vi "MEMR-Initialize Analysis.vi"(0 "Expt State":T3, 5 "Params":T5, 11 "error in (no error)":errorcluster, 13 "controls":T4) -> (4 "State":T1, 8 "Analysis":T2, 15 "error out":errorcluster)   [LabVIEW 2020]
uses:
  Typedefs/MEMR-Params.ctl
  Typedefs/MEMR-Probe.ctl
  Typedefs/MEMR-Elicitor.ctl
  Human Studies/SFM Frontend/LV Source/Typedefs/HSTS-Transducer.ctl
  Typedefs/MEMR-Sequence.ctl
  Typedefs/MEMR-Analysis.ctl
  Typedefs/MEMR-Timing.ctl
  Typedefs/MEMR-Controls.ctl
  CFTS Main Panel SubVIs/CFTS-Experiment State.ctl
  Typedefs/MEMR-Analysis State.ctl
  Utility VIs/Math VIs/dB to Linear (scalar).vi
  Utility VIs/Math VIs/LinSpace (start-stop-step).vi
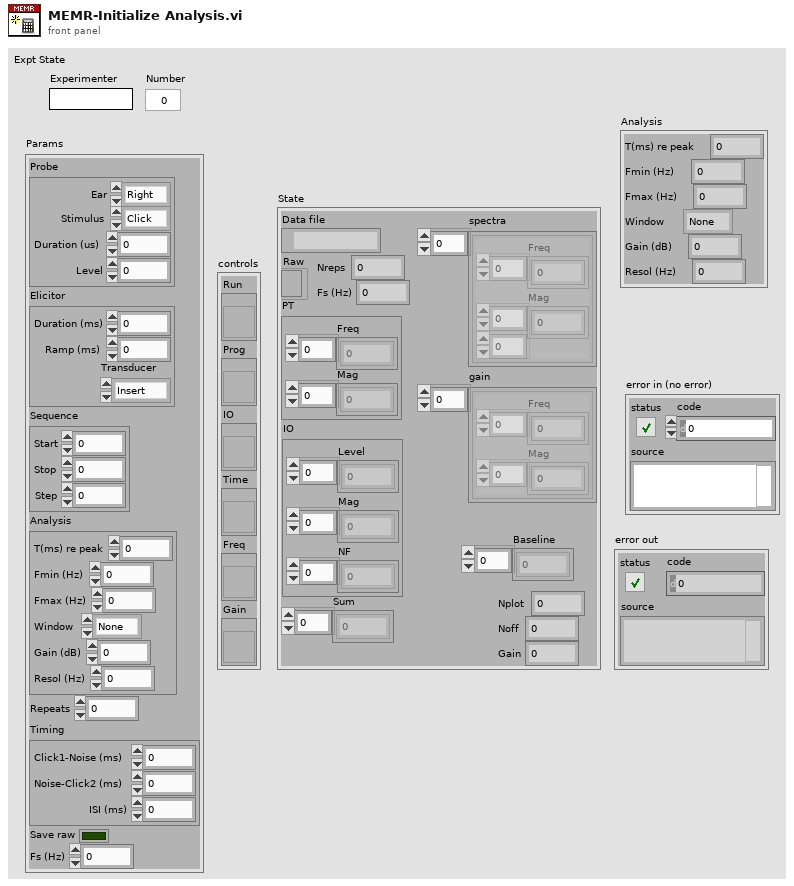
[diagram p1: front panel]
types:
  T1 = typedef "MEMR-Analysis State.ctl" = cluster{"Data file":path, "Raw":refnum<file>, "PT":cluster{"Freq":dbl[], "Mag":dbl[]}, "IO":cluster{"Level":dbl[], "Mag":dbl[], "NF":dbl[]}, "Nreps":i32, "Fs (Hz)":dbl, "Sum":dbl[], "Nplot":i32, "Noff":i32, "Gain":dbl, "spectra":cluster{"Freq":dbl[], "Mag":dbl[][]}[], "gain":cluster{"Freq":dbl[], "Mag":dbl[]}[], "Baseline":dbl[]}
  T2 = typedef "MEMR-Analysis.ctl" = cluster{"T(ms) re peak":dbl, "Fmin (Hz)":dbl, "Fmax (Hz)":dbl, "Window":enum16{"None", "Hanning", "Hamming"}, "Gain (dB)":dbl, "Resol (Hz)":dbl}
  T3 = typedef "CFTS-Experiment State.ctl" = cluster{"Experimenter":string, "Number":u32, "Right":string, "Left":string, "Data Folder":path, "State File":path, "Version Info":string, "End Exposure Time":dbl, "Exposure Duration":string, "Run #":cluster{"CAP":i16, "ABR":i16, "DP":i16, "VsEP":i16, "MeasSeq":i16, "SubSeq":i16, "SFOAE":i16}}
  T4 = typedef "MEMR-Controls.ctl" = cluster{"Run":refnum<vi>, "Prog":refnum<vi>, "IO":refnum<vi>, "Time":refnum<vi>, "Freq":refnum<vi>, "Gain":refnum<vi>}
  T5 = typedef "MEMR-Params.ctl" = cluster{"Probe":T6, "Elicitor":T7, "Sequence":T9, "Analysis":T2, "Repeats":i32, "Timing":T10, "Save raw":bool, "Fs (Hz)":dbl}
  T6 = typedef "MEMR-Probe.ctl" = cluster{"Ear":enum16{"Right", "Left"}, "Stimulus":enum16{"Click", "Chirp"}, "Duration (us)":dbl, "Level":dbl}
  T7 = typedef "MEMR-Elicitor.ctl" = cluster{"Duration (ms)":dbl, "Ramp (ms)":dbl, "Transducer":T8}
  T8 = typedef "HSTS-Transducer.ctl" = enum16{"Insert", "TDH-39", "HD300", "ER-10X"}
  T9 = typedef "MEMR-Sequence.ctl" = cluster{"Start":dbl, "Stop":dbl, "Step":dbl}
  T10 = typedef "MEMR-Timing.ctl" = cluster{"Click1-Noise (ms)":dbl, "Noise-Click2 (ms)":dbl, "ISI (ms)":dbl}
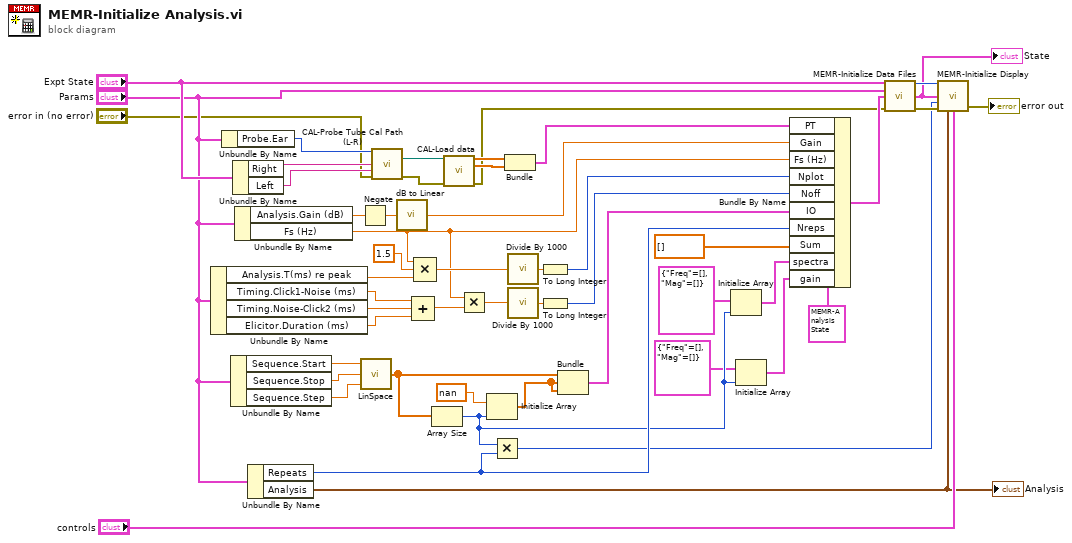
[diagram p0: block diagram]
diagram:
  n1 = Unbundle By Name("Params") -> ("Analysis.T(ms) re peak"=w25:dbl, "Timing.Click1-Noise (ms)"=w20:dbl, "Timing.Noise-Click2 (ms)"=w19:dbl, "Elicitor.Duration (ms)"=w18:dbl)
  n2 = Unbundle By Name("Params") -> ("Probe.Ear"=w48:enum16{"Right", "Left"})
  n3 = Unbundle By Name("Params") -> ("Sequence.Start"=w42:dbl, "Sequence.Stop"=w40:dbl, "Sequence.Step"=w41:dbl)
  n4 = Unbundle By Name("Expt State") -> ("Right"=w50:string, "Left"=w49:string)
  n5 = Unbundle By Name("Params") -> ("Analysis.Gain (dB)"=w9:dbl, "Fs (Hz)"=w15:dbl)
  n6 = Unbundle By Name("Params") -> ("Repeats"=w35:i32, "Analysis"=w26:T2)
  "Analysis" <- w26
  n7 = Negate(x=w9) -> (-x=w8:dbl)
  n8 = call-poly "LinSpace.vi"("Step"=w41, "Stop"=w40, "Start"=w42) -> ("Array"=w38:dbl[])  [unwired: 1 in, 1 out]
  n9 = call "CAL-Probe Tube Cal Path (L-R).vi"("Ear"=w48, "Right"=w50, "Left"=w49, "error in (no error)"="error in (no error)") -> ("Probe Tube Cal Path"=w47:path, "error out"=w46:errorcluster)  [unwired: 10 in]
  n10 = call-poly "dB to Linear.vi"("dB"=w8) -> ("linear"=w7:dbl)
  n11 = Compound Arithmetic op=ADD(w20, w19, w18) -> (w17:dbl)
  n12 = Compound Arithmetic op=MULTIPLY(w15, 1.5 ("x"), w25) -> (w22:dbl)
  n13 = Array Size(array=w38) -> (size(s)=w3:i32)
  n14 = call "CAL-Load data.vi"("user path"=w47, "error in (no error)"=w46) -> ("Frequency (Hz)"=w45:dbl[], "Mag"=w44:dbl[], "error out"=w11:errorcluster)  [unwired: 6 in, 5 out]
  n15 = Multiply(x=w15, y=w17) -> (x*y=w14:dbl)
  n16 = Initialize Array(nan, w3) -> (w5:dbl[])
  n17 = Multiply(x=w3, y=w35) -> (x*y=w30:i32)
  n18 = Bundle("Frequency (Hz)"=w45, "Mag"=w44) -> (w43:cluster{"Frequency (Hz)":dbl[], "Mag":dbl[]})  [unwired: 1 in]
  n19 = call "Divide By 1000.vi"("X"=w22) -> ("X/1000"=w16:dbl)
  n20 = call "Divide By 1000.vi"("X"=w14) -> ("X/1000"=w13:dbl)
  n21 = To Long Integer(number=w16) -> (32bit integer=w21:i32)
  n22 = To Long Integer(number=w13) -> (32bit integer=w12:i32)
  n23 = Bundle("Array"=w38, w5, w5) -> (w37:cluster{"Array":dbl[], dbl[], dbl[]})  [unwired: 1 in]
  n24 = Initialize Array(cluster{"Freq":dbl[], "Mag":dbl[][]} {"Freq"=[], "Mag"=[]} ("spectra"), w3) -> (w4:cluster{"Freq":dbl[], "Mag":dbl[][]}[])
  n25 = Initialize Array(cluster{"Freq":dbl[], "Mag":dbl[]} {"Freq"=[], "Mag"=[]} ("spectra"), w3) -> (w1:cluster{"Freq":dbl[], "Mag":dbl[]}[])
  n26 = Bundle By Name(cluster=T1 {"Data file"=path "", "Raw"=refnum, "PT"={"Freq"=[], "Mag"=[]}, "IO"={"Level"=[], "Mag"=[], "NF"=[]}, "Nreps"=0, "Fs (Hz)"=0.0, "Sum"=[], "Nplot"=0, "Noff"=0, "Gain"=0.0, "spectra"=[], "gain"=[], "Baseline"=[]} ("Analysis State"), "PT"=w43, "Gain"=w7, "Fs (Hz)"=w15, "Nplot"=w21, "Noff"=w12, "IO"=w37, "Nreps"=w35, "Sum"=dbl[] [] ("Avg"), "spectra"=w4, "gain"=w1) -> (w34:T1)
  n27 = call "MEMR-Initialize Data Files.vi"("Expt State"="Expt State", "Params"="Params", "State In"=w34, "error in (no error)"=w11) -> ("Run"=w28:i32, "State Out"=w27:T1, "error out"=w32:errorcluster)  [unwired: 9 in]
  "State" <- w27
  n28 = call "MEMR-Initialize Display.vi"("Run"=w28, "State"=w27, "Total Nreps"=w30, "error in (no error)"=w32, "Analysis"=w26, "controls"="controls") -> ("error out"=→"error out":errorcluster)  [unwired: 9 in]
